vi "Signal.Export.StringArray.vi"(11 "Signal Parameters":T1 {"Byte Order" items=["Little Endian", "Big Endian"]; "Data Type" items=["Signed", "Unsigned", "IEEE Float"]}) -> (3 "Array":string[](array[string]))   [LabVIEW 2019, in "Diagnostics Addon System Explorer.lvlib"]
uses:
  Diagnostics Addon System Explorer.lvlib
  Addon Shared/Types/Signal.ctl
  Addon Shared/Diagnostics Addon Shared.lvlib
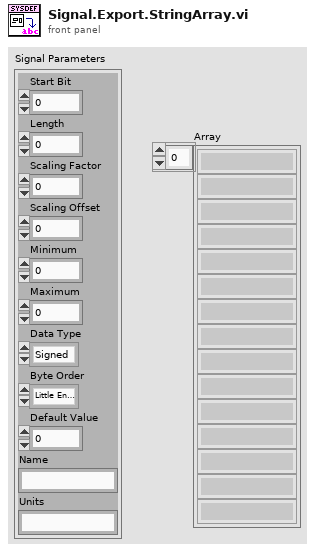
[diagram p1: front panel]
types:
  T1 = typedef "Diagnostics Addon Shared.lvlib/Signal.ctl" = cluster{"Start Bit":u32, "Length":u32, "Scaling Factor":dbl, "Scaling Offset":dbl, "Minimum":dbl, "Maximum":dbl, "Data Type":u32, "Byte Order":u32, "Default Value":dbl, "Name":string, "Units":string}
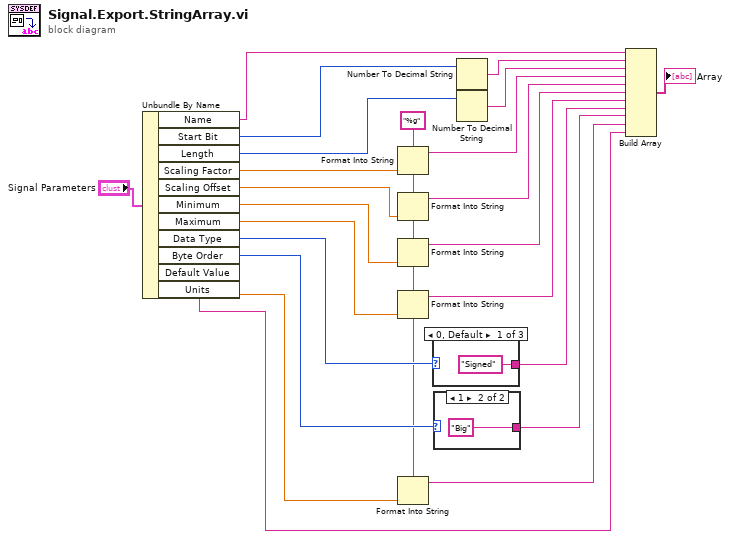
[diagram p0: block diagram]
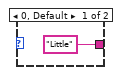
[diagram p2: hidden frame]
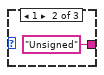
[diagram p3: hidden frame]
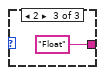
[diagram p4: hidden frame]
diagram:
  w1 = "%g" ("format string")
  n1 = Unbundle By Name("Signal Parameters") -> ("Name"=w19:string, "Start Bit"=w18:u32, "Length"=w17:u32, "Scaling Factor"=w11:dbl, "Scaling Offset"=w3:dbl, "Minimum"=w5:dbl, "Maximum"=w9:dbl, "Data Type"=w16:u32, "Byte Order"=w14:u32, "Default Value"=w7:dbl, "Units"=w12:string)
  n2 = Format Into String(format string=w1, w11) -> (resulting string=w10:string)  [unwired: 2 in, 1 out]
  n3 = Format Into String(format string=w1, w3) -> (resulting string=w2:string)  [unwired: 2 in, 1 out]
  n4 = Format Into String(format string=w1, w5) -> (resulting string=w4:string)  [unwired: 2 in, 1 out]
  n5 = Format Into String(format string=w1, w9) -> (resulting string=w8:string)  [unwired: 2 in, 1 out]
  n6 = Format Into String(format string=w1, w7) -> (resulting string=w6:string)  [unwired: 2 in, 1 out]
  n7 = case shown="0, Default" w16 {
    tunnel: ["Signed" "Unsigned" "Float"] -> w15
    frame 0, Default {
    }
    frame 1 {
    }
    frame 2 {
    }
  }
  n8 = case shown="1" w14 {
    tunnel: ["Little" "Big"] -> w13
    frame 0, Default {
    }
    frame 1 {
    }
  }
  n9 = Number To Decimal String(number=w18) -> (decimal integer string=w20:string)  [unwired: 1 in]
  n10 = Number To Decimal String(number=w17) -> (decimal integer string=w21:string)  [unwired: 1 in]
  n11 = Build Array(w19, w20, w21, w10, w2, w4, w8, w15, w13, w6, w12) -> (→"Array":string[])
